vi "Edge List to Graph.vi"(8 "error in (no error)":errorcluster, 10 "Edge List (src: dst0 dst1..dtsn-1)":string[](array[string]), 11 "Graph in":refnum<class "Graph.lvclass">) -> (0 "error out":errorcluster, 3 "Graph out":refnum<class "Graph.lvclass">)   [LabVIEW 2025, in "AOC.lvlib" / "Graph.lvlib" / "Graph.lvclass"]
uses:
  Graph.lvclass
  <vilib>/Utility/miscctls.llb/LVMapReplaceAction.ctl
  Graph.lvclass/Graph.ctl
  b1304c02-141d-4285-8267-50e68906af43.vi
  <vilib>/Utility/error.llb/Trim Whitespace One-Sided.vi
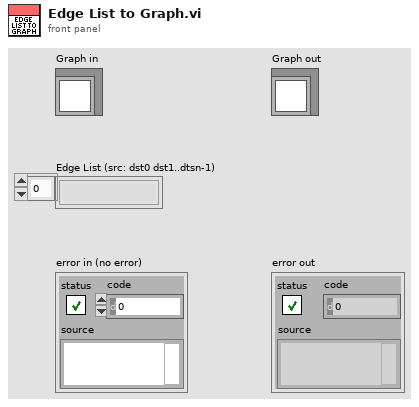
[diagram p1: front panel]
types:
  T1 = typedef "LVMapReplaceAction.ctl" = enum32{"Modify Entry only if found", "Add or Modify Entry", "Delete Entry"}
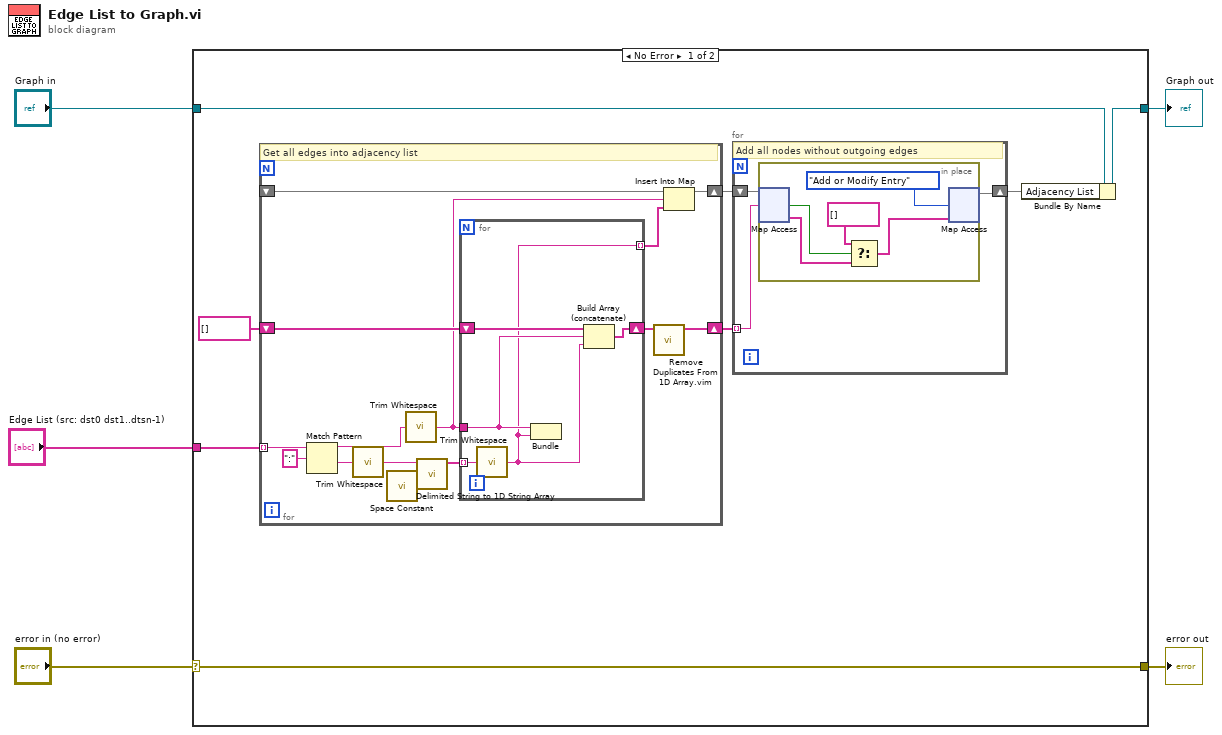
[diagram p0: block diagram]
diagram:
  n1 = case shown="No Error" "error in (no error)" {
    selector: "error in (no error)" -> [w12 w42]
    tunnel: [w12 w42] -> w4
    tunnel: [w11 w41] -> w2
    tunnel: "Graph in" -> [w13 w41]
    tunnel: "Edge List (src: dst0 dst1..dtsn-1)" -> [w10 _]
    frame No Error {
      n2 = for {
        tunnel: w10 -> [w34] mode=indexing
        shift-right: [w29] -> w9
        shift-left: _ -> [w35]
        shift-right: [w22] -> w8
        shift-left: string[] [] ("array with duplicates removed") -> [w27]
        # "Get all edges into adjacency list"
        n3 = Match Pattern(string=w34, regular expression=":" ("search string/char (-)")) -> (before substring=w28:string, after substring=w24:string)  [unwired: 1 in, 2 out]
        n4 = call <vilib>:"Trim Whitespace.vi"("string"=w24) -> ("trimmed string"=w23:string)  [unwired: 1 in]
        n5 = call <vilib>:"Space Constant.vi"() -> ("String"=w32:string)
        n6 = call <vilib>:"Trim Whitespace.vi"("string"=w28) -> ("trimmed string"=w25:string)  [unwired: 1 in]
        n7 = call <vilib>:"Delimited String to 1D String Array.vi"("delimiter"=w32, "delimited string"=w23) -> ("string array"=w31:string[])  [unwired: 9 in]
        n8 = for {
          tunnel: w31 -> [w40] mode=indexing
          tunnel: [w36] -> w30 mode=indexing
          tunnel: w25 -> [w37]
          shift-right: [w38] -> w26
          shift-left: w27 -> [w39]
          n9 = call <vilib>:"Trim Whitespace.vi"("string"=w40) -> ("trimmed string"=w36:string)  [unwired: 1 in]
          n10 = Bundle("trimmed string"=w37, "trimmed string"=w36) -> ()  [unwired: 1 in, 1 out]
          n11 = Build Array (concatenate)(w39, w37, w36) -> (w38:string[])
        }
        n12 = call "Remove Duplicates From 1D Array.vim"("array"=w26) -> ("array with duplicates removed"=w22:string[])  [unwired: 10 in]
        n13 = Insert Into Map(map in=w35, key=w25, value=w30) -> (map out=w29:map{string, string[]})  [unwired: 2 out]
      }
      n14 = for {
        shift-right: [w14] -> w6
        shift-left: w9 -> [w16]
        tunnel: w8 -> [w15] mode=indexing
        # "Add all nodes without outgoing edges"
        n15 = in-place {
          n16 = in-place-map #1(w16, w15) -> (w19:string[], w20:bool)  [unwired: 1 in]
          n17 = Select(t=string[] [], s=w20, f=w19) -> (s? t:f=w17:string[])
          n18 = in-place-map #1(w17, LVMapReplaceAction."Add or Modify Entry" ("action")) -> (w14:map{string, string[]})  [unwired: 2 out]
        }
      }
      n19 = Bundle By Name(cluster=w13, "Adjacency List"=w6) -> (w11:refnum<class "Graph.lvclass">)
    }
    frame Error {
    }
  }
  "error out" <- w4
  "Graph out" <- w2
